vi "Notify Generic Message Event Complete.vi"(8 "error in (no error)":errorcluster, 9 "Response":string, 10 "Completion Id":i64, 11 "Session in":refnum<class "Plugin Session.lvclass">) -> (0 "error out":errorcluster, 3 "Session out":refnum<class "Plugin Session.lvclass">)   [LabVIEW 2021, in "InstrumentStudio Plugin SDK.lvlib" / "Plugin Session.lvclass"]
doc: "Call this VI to notify the framework that the Generic Message event is complete. It is critical that the 'Notify Generic Message Event Complete.vi' is called in the Generic Message event so the framework does not hang"
uses:
  Plugin Session.lvclass
  Plugin Session.lvclass/Plugin Session.ctl
  Read Session Id.vi
  NationalInstruments.VIHost.Interop.dll
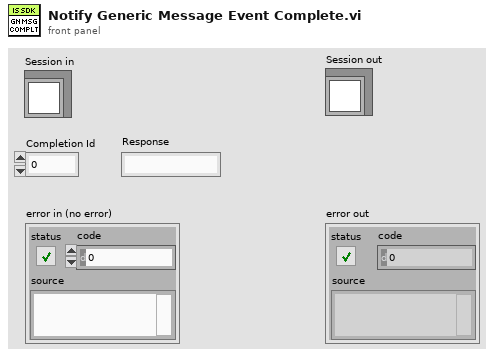
[diagram p1: front panel]
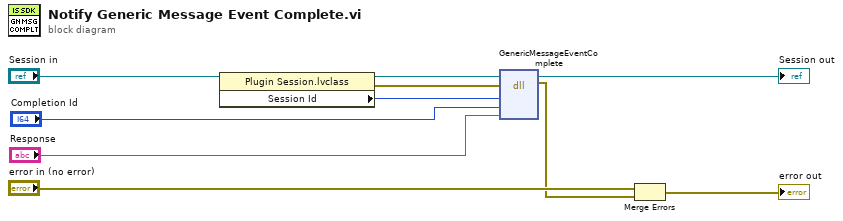
[diagram p0: block diagram]
diagram:
  n1 = property class="Plugin Session.lvclass"(reference="Session in") -> (reference out=→"Session out":refnum<class "Plugin Session.lvclass">, error out=w6:errorcluster, "Session Id"=w5:u64)  [unwired: 1 in]
  n2 = dll-call lib="C:/git/srd-adg-rf/dst/dstd/DSTInstStudio/source/utilities/PluginSDK/NationalInstruments.VIHost.Interop.dll" fn="GenericMessageEventComplete"(error in=w6, "hostId"=w5, "completionId"="Completion Id", "response"="Response") -> (error out=w3:errorcluster)  [unwired: 6 in, 1 out]
  n3 = Merge Errors("error in (no error)", w3) -> (→"error out":errorcluster)
